vi "export_data.vi"(10 "vacuum":sgl, 11 "index":i32) -> ()   [LabVIEW 2012]
uses:
  FT_HMI.llb/GLOBAL_PUMPS_PARAMS.vi
  FT_HMI.llb/GLOBAL_GEN.vi
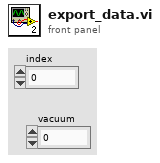
[diagram p1: front panel]
types:
  T1 = cluster{"VAC":cluster{"ENABLE":bool, "PUMPING_TIME [ms]":dbl, "MEASUREMENT_TIME [ms]":dbl, "PRESSURE_LIMIT [bar]":sgl}, "Q1":cluster{"ENABLE":bool, "PUMPING_TIME  [ms]":dbl, "MEASUREMENT_TIME  [ms]":sgl, "FLOW_TARGET  [ml/min]":sgl, "FLOW_LIMIT_UP  [ml/min]":sgl, "FLOW_LIMIT_DOWN [ml/min]":sgl, "PRESSURE_TARGET [bar]":sgl, "PRESSURE_LIMIT_UP [bar]":sgl, "PRESSURE_LIMIT_DOWN [bar]":sgl, "MAX_FLOW":bool}, "Q2":cluster{"ENABLE":bool, "PUMPING_TIME [ms]":dbl, "MEASUREMENT_TIME [ms]":dbl, "FLOW_TARGET [ml/min]":sgl, "FLOW_LIMIT_UP [ml/min]":sgl, "FLOW_LIMIT_DOWN [ml/min]":sgl, "PRESSURE_TARGET [bar]":sgl, "PRESSURE_LIMIT_UP [bar]":sgl, "PRESSURE_LIMIT_DOWN [bar]":sgl, "MAX_FLOW":bool}, "PMAX":cluster{"ENABLE":bool, "PUMPING_TIME [ms]":dbl, "MEASUREMENT_TIME [ms]":dbl, "PRESSURE_LIMIT [bar]":sgl, "PRESSURE_LOOSE_TIME [ms]":sgl}, "PRINT":cluster{"ENABLE":bool}, "SUPPLY":cluster{"VOLTAGE [V]":dbl, "FREQUENCY [Hz]":dbl}}
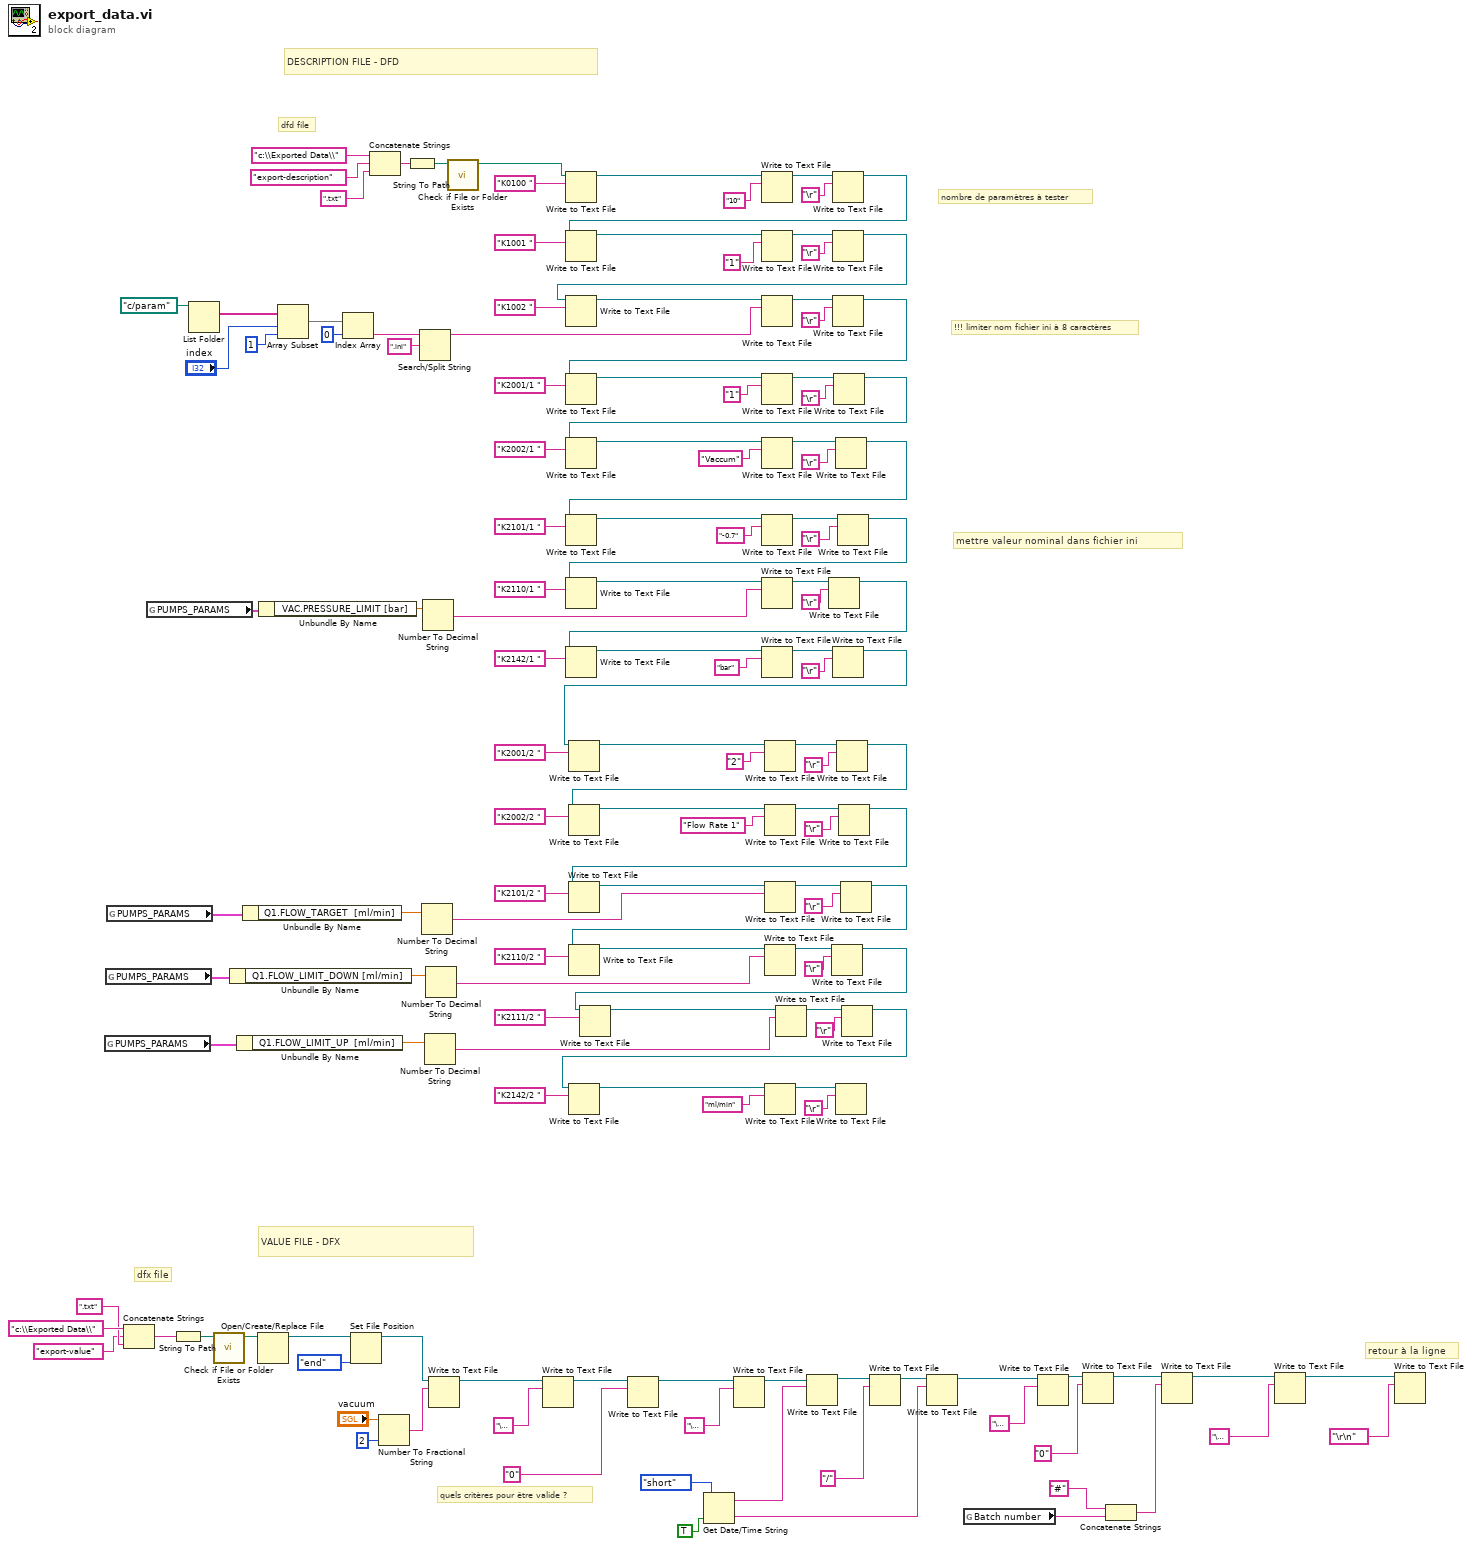
[diagram p0: block diagram]
diagram:
  # "dfx file"
  # "VALUE FILE - DFX"
  # "DESCRIPTION FILE - DFD"
  # "dfd file"
  # "quels critères pour être valide ?"
  # "!!! limiter nom fichier ini à 8 caractères"
  # "nombre de paramètres à tester"
  # "mettre valeur nominal dans fichier ini"
  # "retour à la ligne"
  n1 = global read "GLOBAL_PUMPS_PARAMS.vi" "PUMPS_PARAMS"() -> (w13:T1)
  n2 = global read "GLOBAL_PUMPS_PARAMS.vi" "PUMPS_PARAMS"() -> (w45:T1)
  n3 = global read "GLOBAL_PUMPS_PARAMS.vi" "PUMPS_PARAMS"() -> (w16:T1)
  n4 = Concatenate Strings("c:\\Exported Data\\", "export-value" ("string"), ".txt") -> (w77:string)
  n5 = global read "GLOBAL_PUMPS_PARAMS.vi" "PUMPS_PARAMS"() -> (w121:T1)
  n6 = String To Path(string=w77) -> (path=w79:path)
  n7 = List Folder(path=path "c:/param") -> (filenames=w119:string[])  [unwired: 3 in, 3 out]
  n8 = call <vilib>:"Check if File or Folder Exists.vi"("path"=w79) -> ("dup path"=w49:path)  [unwired: 8 in, 2 out]
  n9 = Unbundle By Name(w45) -> ("Q1.FLOW_LIMIT_DOWN [ml/min]"=w23:sgl)
  n10 = Unbundle By Name(w13) -> ("Q1.FLOW_LIMIT_UP  [ml/min]"=w12:sgl)
  n11 = Unbundle By Name(w16) -> ("Q1.FLOW_TARGET  [ml/min]"=w15:sgl)
  n12 = Open/Create/Replace File(file path (use dialog)=w49) -> (refnum out=w47:refnum<file>)  [unwired: 5 in, 2 out]
  n13 = Unbundle By Name(w121) -> ("VAC.PRESSURE_LIMIT [bar]"=w88:sgl)
  n14 = Array Subset(array=w119, index="index", length=1) -> (w112:string[])
  n15 = Index Array(array=w112, index=0) -> (element=w100:string)
  n16 = Set File Position(refnum=w47, from (0:start)=enum16{"start", "end", "current"}."end") -> (refnum out=w46:refnum<file>)  [unwired: 2 in, 1 out]
  n17 = Concatenate Strings("c:\\Exported Data\\", "export-description" ("string"), ".txt") -> (w140:string)
  n18 = Number To Fractional String(number="vacuum", precision (6)=i16 2 ("width (-)")) -> (F-format string=w50:string)  [unwired: 2 in]
  n19 = String To Path(string=w140) -> (path=w142:path)
  n20 = Search/Split String(string=w100, search string/char (-)=".ini") -> (substring before match=w102:string)  [unwired: 1 in, 2 out]
  n21 = Number To Decimal String(number=w15) -> (decimal integer string=w14:string)  [unwired: 1 in]
  n22 = Number To Decimal String(number=w88) -> (decimal integer string=w87:string)  [unwired: 1 in]
  n23 = Number To Decimal String(number=w12) -> (decimal integer string=w7:string)  [unwired: 1 in]
  n24 = Number To Decimal String(number=w23) -> (decimal integer string=w22:string)  [unwired: 1 in]
  n25 = Write to Text File(file (use dialog)=w46, text=w50) -> (refnum out=w75:refnum<file>)  [unwired: 2 in, 2 out]
  n26 = call <vilib>:"Check if File or Folder Exists.vi"("path"=w142) -> ("dup path"=w137:path)  [unwired: 8 in, 2 out]
  n27 = Write to Text File(file (use dialog)=w75, text="\u0014") -> (refnum out=w72:refnum<file>)  [unwired: 2 in, 2 out]
  n28 = Write to Text File(file (use dialog)=w137, text="K0100 ") -> (refnum out=w135:refnum<file>)  [unwired: 2 in, 2 out]
  n29 = Write to Text File(file (use dialog)=w72, text="0") -> (refnum out=w71:refnum<file>)  [unwired: 2 in, 2 out]
  n30 = Get Date/Time String(date format (0)=enum16{"short", "long", "abbreviated"}."short", want seconds? (F)=TRUE) -> (date string=w67:string, time string=w66:string)  [unwired: 1 in]
  n31 = Write to Text File(file (use dialog)=w71, text="\u0014") -> (refnum out=w68:refnum<file>)  [unwired: 2 in, 2 out]
  n32 = Write to Text File(file (use dialog)=w135, text="10") -> (refnum out=w134:refnum<file>)  [unwired: 2 in, 2 out]
  n33 = Write to Text File(file (use dialog)=w68, text=w67) -> (refnum out=w63:refnum<file>)  [unwired: 2 in, 2 out]
  n34 = Write to Text File(file (use dialog)=w134, text="\r") -> (refnum out=w127:refnum<file>)  [unwired: 2 in, 2 out]
  n35 = Write to Text File(file (use dialog)=w127, text="K1001 ") -> (refnum out=w130:refnum<file>)  [unwired: 2 in, 2 out]
  n36 = Write to Text File(file (use dialog)=w130, text="1") -> (refnum out=w129:refnum<file>)  [unwired: 2 in, 2 out]
  n37 = Write to Text File(file (use dialog)=w129, text="\r") -> (refnum out=w122:refnum<file>)  [unwired: 2 in, 2 out]
  n38 = Write to Text File(file (use dialog)=w122, text="K1002 ") -> (refnum out=w125:refnum<file>)  [unwired: 2 in, 2 out]
  n39 = Write to Text File(file (use dialog)=w125, text=w102) -> (refnum out=w124:refnum<file>)  [unwired: 2 in, 2 out]
  n40 = Write to Text File(file (use dialog)=w124, text="\r") -> (refnum out=w114:refnum<file>)  [unwired: 2 in, 2 out]
  n41 = Write to Text File(file (use dialog)=w114, text="K2001/1 ") -> (refnum out=w117:refnum<file>)  [unwired: 2 in, 2 out]
  n42 = Write to Text File(file (use dialog)=w117, text="1") -> (refnum out=w116:refnum<file>)  [unwired: 2 in, 2 out]
  n43 = Write to Text File(file (use dialog)=w116, text="\r") -> (refnum out=w104:refnum<file>)  [unwired: 2 in, 2 out]
  n44 = Write to Text File(file (use dialog)=w104, text="K2002/1 ") -> (refnum out=w108:refnum<file>)  [unwired: 2 in, 2 out]
  n45 = Write to Text File(file (use dialog)=w108, text="Vaccum") -> (refnum out=w107:refnum<file>)  [unwired: 2 in, 2 out]
  n46 = Write to Text File(file (use dialog)=w107, text="\r") -> (refnum out=w90:refnum<file>)  [unwired: 2 in, 2 out]
  n47 = Write to Text File(file (use dialog)=w90, text="K2101/1 ") -> (refnum out=w98:refnum<file>)  [unwired: 2 in, 2 out]
  n48 = Write to Text File(file (use dialog)=w98, text="-0.7") -> (refnum out=w97:refnum<file>)  [unwired: 2 in, 2 out]
  n49 = Write to Text File(file (use dialog)=w97, text="\r") -> (refnum out=w89:refnum<file>)  [unwired: 2 in, 2 out]
  n50 = Write to Text File(file (use dialog)=w89, text="K2110/1 ") -> (refnum out=w93:refnum<file>)  [unwired: 2 in, 2 out]
  n51 = Write to Text File(file (use dialog)=w93, text=w87) -> (refnum out=w92:refnum<file>)  [unwired: 2 in, 2 out]
  n52 = Write to Text File(file (use dialog)=w92, text="\r") -> (refnum out=w81:refnum<file>)  [unwired: 2 in, 2 out]
  n53 = Write to Text File(file (use dialog)=w81, text="K2142/1 ") -> (refnum out=w85:refnum<file>)  [unwired: 2 in, 2 out]
  n54 = Write to Text File(file (use dialog)=w85, text="bar") -> (refnum out=w84:refnum<file>)  [unwired: 2 in, 2 out]
  n55 = Write to Text File(file (use dialog)=w84, text="\r") -> (refnum out=w4:refnum<file>)  [unwired: 2 in, 2 out]
  n56 = Write to Text File(file (use dialog)=w4, text="K2001/2 ") -> (refnum out=w43:refnum<file>)  [unwired: 2 in, 2 out]
  n57 = Write to Text File(file (use dialog)=w43, text="2") -> (refnum out=w42:refnum<file>)  [unwired: 2 in, 2 out]
  n58 = Write to Text File(file (use dialog)=w42, text="\r") -> (refnum out=w34:refnum<file>)  [unwired: 2 in, 2 out]
  n59 = Write to Text File(file (use dialog)=w34, text="K2002/2 ") -> (refnum out=w38:refnum<file>)  [unwired: 2 in, 2 out]
  n60 = Write to Text File(file (use dialog)=w38, text="Flow Rate 1") -> (refnum out=w37:refnum<file>)  [unwired: 2 in, 2 out]
  n61 = Write to Text File(file (use dialog)=w37, text="\r") -> (refnum out=w25:refnum<file>)  [unwired: 2 in, 2 out]
  n62 = Write to Text File(file (use dialog)=w25, text="K2101/2 ") -> (refnum out=w32:refnum<file>)  [unwired: 2 in, 2 out]
  n63 = Write to Text File(file (use dialog)=w32, text=w14) -> (refnum out=w31:refnum<file>)  [unwired: 2 in, 2 out]
  n64 = Write to Text File(file (use dialog)=w31, text="\r") -> (refnum out=w24:refnum<file>)  [unwired: 2 in, 2 out]
  n65 = Write to Text File(file (use dialog)=w24, text="K2110/2 ") -> (refnum out=w28:refnum<file>)  [unwired: 2 in, 2 out]
  n66 = Write to Text File(file (use dialog)=w28, text=w22) -> (refnum out=w27:refnum<file>)  [unwired: 2 in, 2 out]
  n67 = Write to Text File(file (use dialog)=w27, text="\r") -> (refnum out=w6:refnum<file>)  [unwired: 2 in, 2 out]
  n68 = Write to Text File(file (use dialog)=w6, text="K2111/2 ") -> (refnum out=w10:refnum<file>)  [unwired: 2 in, 2 out]
  n69 = Write to Text File(file (use dialog)=w10, text=w7) -> (refnum out=w9:refnum<file>)  [unwired: 2 in, 2 out]
  n70 = Write to Text File(file (use dialog)=w9, text="\r") -> (refnum out=w5:refnum<file>)  [unwired: 2 in, 2 out]
  n71 = Write to Text File(file (use dialog)=w5, text="K2142/2 ") -> (refnum out=w20:refnum<file>)  [unwired: 2 in, 2 out]
  n72 = Write to Text File(file (use dialog)=w20, text="ml/min") -> (refnum out=w19:refnum<file>)  [unwired: 2 in, 2 out]
  n73 = Write to Text File(file (use dialog)=w19, text="\r") -> ()  [unwired: 2 in, 3 out]
  n74 = Write to Text File(file (use dialog)=w63, text="/") -> (refnum out=w62:refnum<file>)  [unwired: 2 in, 2 out]
  n75 = Write to Text File(file (use dialog)=w62, text=w66) -> (refnum out=w65:refnum<file>)  [unwired: 2 in, 2 out]
  n76 = global read "GLOBAL_GEN.vi" "Batch number"() -> (w58:string)
  n77 = Write to Text File(file (use dialog)=w65, text="\u0014") -> (refnum out=w59:refnum<file>)  [unwired: 2 in, 2 out]
  n78 = Write to Text File(file (use dialog)=w59, text="0") -> (refnum out=w56:refnum<file>)  [unwired: 2 in, 2 out]
  n79 = Concatenate Strings("#" ("string"), w58) -> (w55:string)
  n80 = Write to Text File(file (use dialog)=w56, text=w55) -> (refnum out=w54:refnum<file>)  [unwired: 2 in, 2 out]
  n81 = Write to Text File(file (use dialog)=w54, text="\u000f") -> (refnum out=w51:refnum<file>)  [unwired: 2 in, 2 out]
  n82 = Write to Text File(file (use dialog)=w51, text="\r\n") -> ()  [unwired: 2 in, 3 out]
